vi "XMLCloseConfiguration.vi"(8 "error in (no error)":errorcluster, 10 "OPC UA server refnum in":refnum<k21>, 11 "DOM document in":refnum<k20>) -> (0 "error out":errorcluster, 2 "OPC UA server refnum out":refnum<k21>)   [LabVIEW 2014, in "OPCUA XML.lvlib"]
uses:
  OPCUA XML.lvlib
  <vilib>/xml/Close Reference(Node).vi
  <vilib>/xml/NI_XML.lvlib
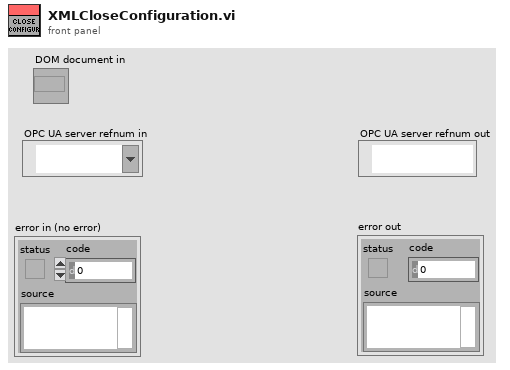
[diagram p1: front panel]
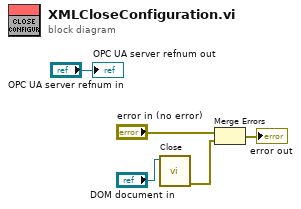
[diagram p0: block diagram]
diagram:
  n1 = call-poly <vilib>:"Close.vi"("node"="DOM document in") -> ("error out"=w4:errorcluster)  [unwired: 1 in, 7 out]
  n2 = Merge Errors("error in (no error)", w4) -> (→"error out":errorcluster)
  "OPC UA server refnum out" <- "OPC UA server refnum in"
